vi "chaosui-crest-cu-get.vi"(0 "handleConnection":T3, 1 "args":string, 2 "cmd submission mode":enum16{"stack", "kill previous"}(ring), 3 "prio":i32=50, 5 "cuname":string, 9 "timeout (10000)":i32=10000, 11 "cmd":string="status", 13 "sched (ms)":i32=100) -> (4 "dev_error":bool, 6 "dev_state":T1, 10 "timestamp":u64, 12 "output out":string, 15 "nok":i32)   [LabVIEW 2012, in "chaosui-crest.lvlib"]
doc: "uint64_t chaos_crest_cu_get(chaos_crest_handle_t h,const char*cuname,char*output,int maxsize);"
uses:
  chaosui-crest.lvlib
  <vilib>/httpClient/ClientHandle.ctl
  <vilib>/httpClient/LabVIEWHTTPClient.lvlib
  ChaosDevState.ctl
panel:
  in  "dev_state 2":enum16{"stop", "init", "deinit", "start"}(ring)
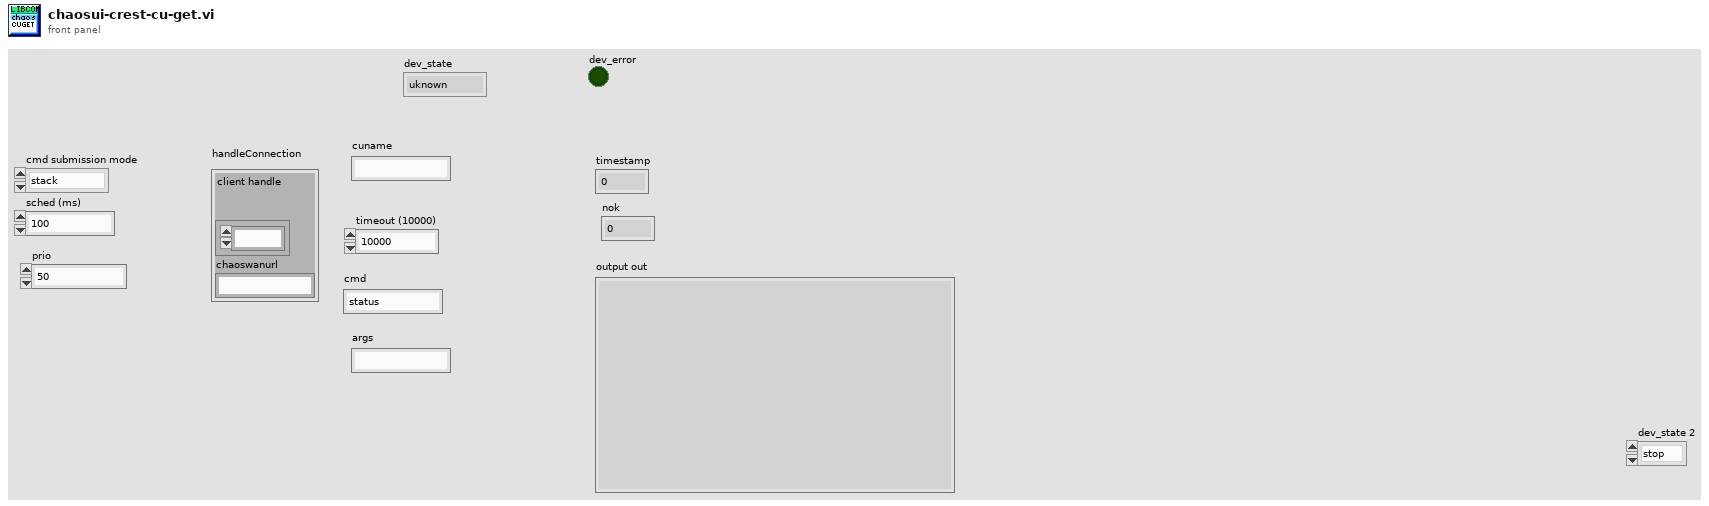
[diagram p1: front panel]
types:
  T1 = typedef "ChaosDevState.ctl" = enum16{"uknown", "stop", "init", "deinit", "start"}
  T2 = typedef "LabVIEWHTTPClient.lvlib/ClientHandle.ctl" = refnum<k1>
  T3 = cluster{"client handle":T2, "chaoswanurl":string}
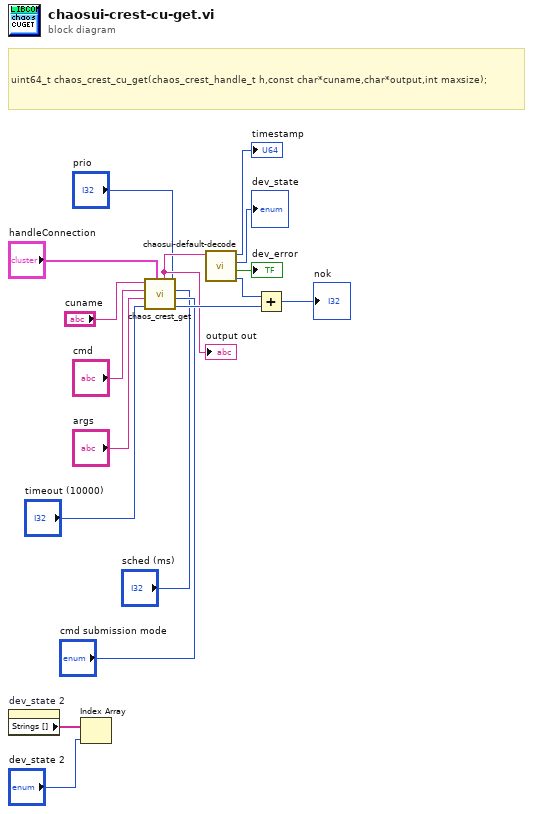
[diagram p0: block diagram]
diagram:
  # "uint64_t chaos_crest_cu_get(chaos_crest_handle_t h,const char*cuname,char*output,int maxsize);"
  n1 = property on="dev_state 2" class="Enum (strict)"() -> ("Strings []"=w12:string[])  [unwired: 2 in, 2 out]
  n2 = Index Array(array=w12, index="dev_state 2") -> ()  [unwired: 1 out]
  n3 = call "chaos_crest_get.vi"("cuname"="cuname", "cmd"="cmd", "args"="args", "timeout (10000)"="timeout (10000)", "handleConnection"="handleConnection", "prio"="prio", "sched (ms)"="sched (ms)", "cmd submission mode"="cmd submission mode") -> ("body"=w8:string, "nok"=w14:i32)  [unwired: 1 out]
  "output out" <- w8
  n4 = call "chaosui-default-decode.vi"("JSON string"=w8) -> ("parse_error"=w6:i32, "dev_error"=→"dev_error":bool, "dev_state"=→"dev_state":T1, "timestamp"=→"timestamp":u64)  [unwired: 3 in, 1 out]
  n5 = Add(x=w6, y=w14) -> (x+y=→"nok":i32)
